vi "Format Notes.vi"(1 "Notes":string) -> (0 "String":string)   [LabVIEW 2016, in "LV to ITX.lvclass"]
uses:
  LV to ITX.lvclass
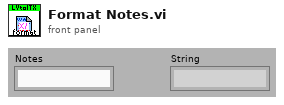
[diagram p1: front panel]
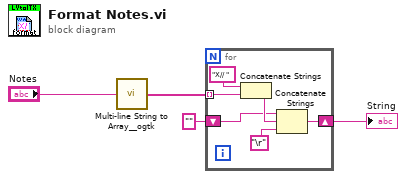
[diagram p0: block diagram]
diagram:
  n1 = call <userlib>:"Multi-line String to Array__ogtk.vi"("string"="Notes") -> ("lines"=w1:string[])
  n2 = for {
    tunnel: w1 -> [w10] mode=indexing
    shift-right: [w8] -> w3
    shift-left: "" -> [w5]
    n3 = Concatenate Strings("X// " ("string"), w10) -> (w7:string)
    n4 = Concatenate Strings(w5, w7, "\r") -> (w8:string)
  }
  "String" <- w3
